vi "SetUp.vi"(8 "error in (no error)":errorcluster, 11 "Prueba10 in":refnum<class "Prueba10.lvclass">) -> (0 "error out":errorcluster, 3 "Prueba10 out":refnum<class "Prueba10.lvclass">)   [LabVIEW 2019, in "Prueba10.lvclass"]
uses:
  Prueba10.lvclass
  Prueba10.lvclass/Prueba10.ctl
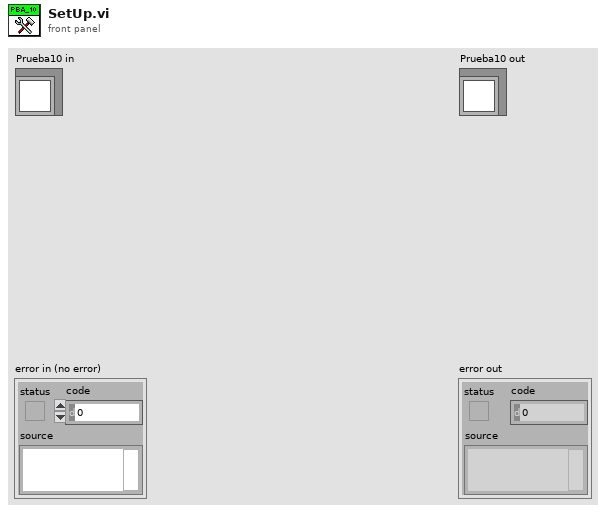
[diagram p1: front panel]
types:
  T1 = typedef "Prueba10.lvclass/BD.ctl" = cluster{"NivMaxMenosSens":dbl, "Incertidumbre":string, "Tol +":string, "Tol -":string}
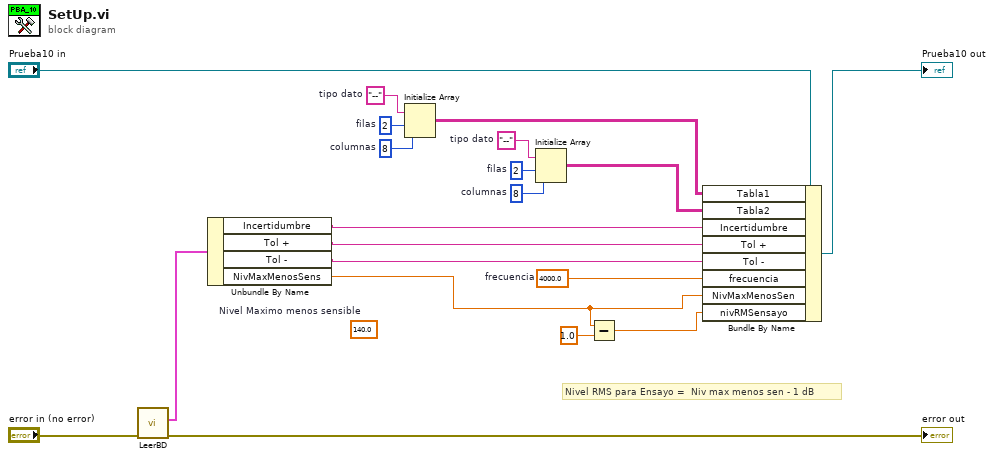
[diagram p0: block diagram]
diagram:
  w9 = 8  # columnas
  w10 = 2  # filas
  w8 = "--"  # tipo dato
  (unwired) 140.0  # Nivel Maximo menos sensible
  w19 = 4000.0  # frecuencia
  w17 = 8  # columnas
  w15 = 2  # filas
  w18 = "--"  # tipo dato
  # "Nivel RMS para Ensayo =  Niv max menos sen - 1 dB"
  n1 = call "LeerBD.vi"("error in (no error)"="error in (no error)") -> ("error out"=→"error out":errorcluster, "BD"=w5:T1)  [unwired: 8 in, 1 out]
  n2 = Unbundle By Name(w5) -> ("Incertidumbre"=w4:string, "Tol +"=w3:string, "Tol -"=w2:string, "NivMaxMenosSens"=w1:dbl)
  n3 = Initialize Array(w8, w10, w9) -> (w7:string[][])
  n4 = Initialize Array(w18, w15, w17) -> (w16:string[][])
  n5 = Subtract(x=w1, y=1.0) -> (x-y=w11:dbl)
  n6 = Bundle By Name(cluster="Prueba10 in", "Tabla1"=w7, "Tabla2"=w16, "Incertidumbre"=w4, "Tol +"=w3, "Tol -"=w2, "frecuencia"=w19, "NivMaxMenosSen"=w1, "nivRMSensayo"=w11) -> (→"Prueba10 out":refnum<class "Prueba10.lvclass">)
